vi "TurnOnRelayArduino.vi"(8 "error in":errorcluster, 9 "channel":i32, 10 "duration":dbl, 11 "LINX Resource":T1) -> (0 "error out":errorcluster, 3 "LINX Resource Out":T1)   [LabVIEW 2015]
uses:
  <vilib>/MakerHub/LINX/Private/Type Defs/LINX Ref.ctl
  <vilib>/MakerHub/LINX/Private/Type Defs/Platform.ctl
  <vilib>/MakerHub/LINX/Private/Type Defs/Interface.ctl
  <vilib>/MakerHub/LINX/Private/Device/Type Defs/LINX Device Config.ctl
  <vilib>/MakerHub/LINX/Private/Device/Type Defs/TCP Config.ctl
  <vilib>/MakerHub/LINX/Private/Device/Type Defs/Channels.ctl
  <vilib>/MakerHub/LINX/Public/Peripherals/PWM/PWM Set Duty Cycle 1 Chan.vi
  <vilib>/MakerHub/LINX/Public/Peripherals/PWM/PWM Set Duty Cycle N Chans.vi
  <vilib>/MakerHub/LINX/LMH-LINX.lvlib
  <vilib>/MakerHub/LINX/Private/Device/Device.lvlib
panel:
  # "Turn on Relay with 5V Analog Signal"
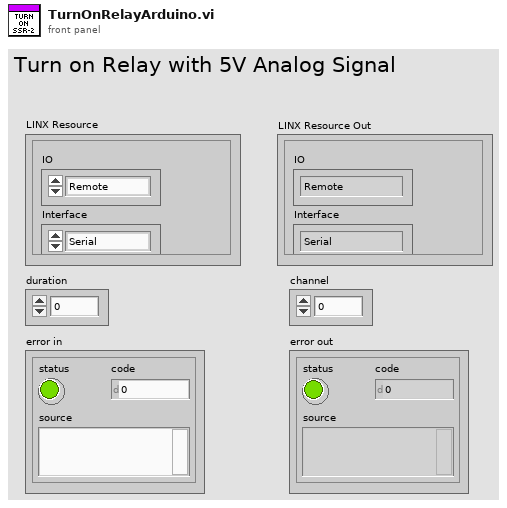
[diagram p1: front panel]
types:
  T1 = typedef "LMH-LINX.lvlib/LINX Ref.ctl" = cluster{"IO":T2, "Interface":T3, "LINX Device Config":T4}
  T2 = typedef "LMH-LINX.lvlib/Platform.ctl" = enum16{"Remote", "Local"}
  T3 = typedef "LMH-LINX.lvlib/Interface.ctl" = enum16{"Serial", "TCP"}
  T4 = typedef "LMH-LINX.lvlib/Device.lvlib/LINX Device Config.ctl" = cluster{"Interface":T3, "COM Port":refnum<visa-resource-name>, "TCP Configuration":T5, "Device Family":u8, "Device ID":u8, "Device Name":string, "TCP Ref":refnum<k5>, "Channels":T6}
  T5 = typedef "LMH-LINX.lvlib/Device.lvlib/TCP Config.ctl" = cluster{"IP Address":string, "Port":u16}
  T6 = typedef "LMH-LINX.lvlib/Channels.ctl" = cluster{"DI":u8[], "DO":u8[], "AI":u8[], "AO":u8[], "PWM":u8[], "QE":u8[], "UART":u8[], "I2C 2":u8[], "SPI":u8[], "CAN":u8[], "Servo":u8[], "AI Ref (V)":dbl, "AI Resolution (Bits)":u8, "AO Ref (V)":dbl, "AO Resolution (Bits)":u8}
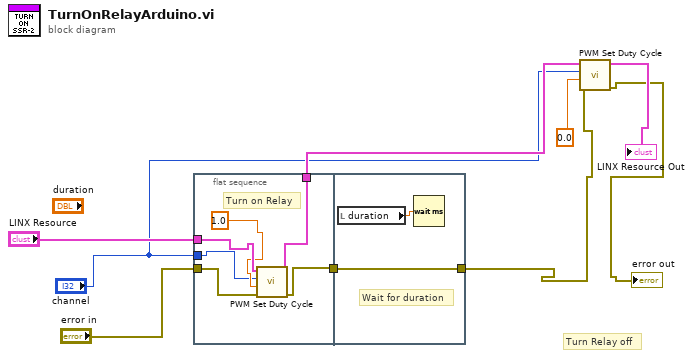
[diagram p0: block diagram]
diagram:
  # "Turn Relay off"
  n1 = flat-sequence {
    tunnel: "error in" -> [w12]
    tunnel: [w15] -> w9
    tunnel: "channel" -> [w10]
    tunnel: "LINX Resource" -> [w13]
    tunnel: [w14] -> w5
    tunnel: [w17] -> w3
    tunnel: w9 -> [w17]
    frame #0 {
      # "Turn on Relay"
      n2 = call-poly <vilib>:"PWM Set Duty Cycle.vi"("Error In"=w12, "Duty Cycle (0-1)"=1.0, "PWM Channel"=w10, "LINX Resource"=w13) -> ("Error Out"=w15:errorcluster, "LINX Resource"=w14:T1)  [unwired: 6 in]
    }
    frame #1 {
      # "Wait for duration"
      n3 = local read "duration"() -> (w16:dbl)
      n4 = Wait (ms)(milliseconds to wait=w16) -> ()  [unwired: 1 out]
    }
  }
  n5 = call-poly <vilib>:"PWM Set Duty Cycle.vi"("Error In"=w3, "Duty Cycle (0-1)"=0.0, "PWM Channel"="channel", "LINX Resource"=w5) -> ("Error Out"=→"error out":errorcluster, "LINX Resource"=→"LINX Resource Out":T1)  [unwired: 6 in]
